vi "AlliGator Load Piccolo hist .bin Data.vi"(4 "# Pixels Y":i32, 6 "# Pixels X":i32, 8 "error in (no error)":errorcluster, 9 "# TCSPC Bins":i32, 11 "path in":path) -> (0 "error out":errorcluster, 2 "Array":u16[][][](array[numeric]), 3 "path out":path)   [LabVIEW 2021, in "AlliGator Files.lvlib"]
doc: "Loads Piccolo binned data."
uses:
  AlliGator Files.lvlib
panel:
  # "see the AlliGator License on the block diagram (Ctrl+E or Window:Show Block Diagram)"
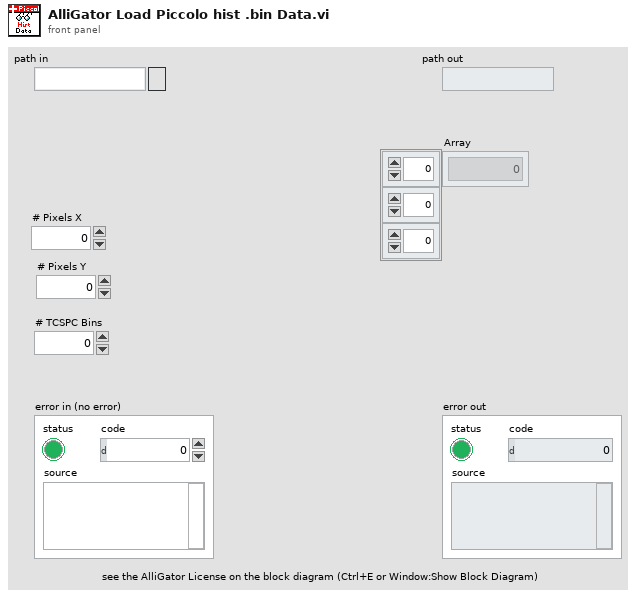
[diagram p1: front panel]
types:
  T1 = enum16{"big-endian, network order", "native, host order", "little-endian"}
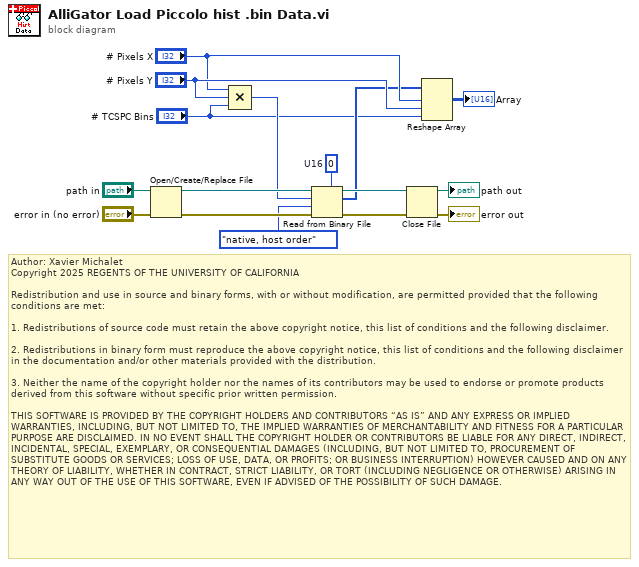
[diagram p0: block diagram]
diagram:
  w7 = u16 0  # U16
  # "Author: Xavier Michalet\nCopyright 2025 REGENTS OF THE UNIVERSITY OF CALIFORNIA\n\nRedistribution and use in source and binary forms, with or without modification, are permitted provided that the following conditions are met:\n\n1. Redistributions of source code must retain the above copyright notice, this list of conditions and the following disclaimer.\n\n2. Redistributions in binary form must reproduce the above copyright notice, this list of conditions and the following disclaimer in the documentation and/or other materials provided with the distribution.\n\n3. Neither the name of the copyright holder nor the names of its contributors may be used to endorse or promote products derived from this software without specific prior written permission.\n\nTHIS SOFTWARE IS PROVIDED BY THE COPYRIGHT HOLDERS AND CONTRIBUTORS “AS IS” AND ANY EXPRESS OR IMPLIED WARRANTIES, INCLUDING, BUT NOT LIMITED TO, THE IMPLIED WARRANTIES OF MERCHANTABILITY AND FITNESS FOR A PARTICULAR PURPOSE ARE DISCLAIMED. IN NO EVENT SHALL THE COPYRIGHT HOLDER OR CONTRIBUTORS BE LIABLE FOR ANY DIRECT, INDIRECT, INCIDENTAL, SPECIAL, EXEMPLARY, OR CONSEQUENTIAL DAMAGES (INCLUDING, BUT NOT LIMITED TO, PROCUREMENT OF SUBSTITUTE GOODS OR SERVICES; LOSS OF USE, DATA, OR PROFITS; OR BUSINESS INTERRUPTION) HOWEVER CAUSED AND ON ANY THEORY OF LIABILITY, WHETHER IN CONTRACT, STRICT LIABILITY, OR TORT (INCLUDING NEGLIGENCE OR OTHERWISE) ARISING IN ANY WAY OUT OF THE USE OF THIS SOFTWARE, EVEN IF ADVISED OF THE POSSIBILITY OF SUCH DAMAGE."
  n1 = Open/Create/Replace File(file path (use dialog)="path in", error in="error in (no error)") -> (refnum out=w13:refnum<file>, error out=w14:errorcluster)  [unwired: 4 in, 1 out]
  n2 = Compound Arithmetic op=MULTIPLY("# Pixels X", "# Pixels Y", "# TCSPC Bins") -> (w4:i32)
  n3 = Read from Binary File(5:w7, 8:w14, 9:T1."native, host order" ("byte order (0:big-endian, network order)"), 10:w4, 11:w13) -> (0:w2:errorcluster, 2:w5:u16[], 3:w15:refnum<file>)  [unwired: 1 in, 1 out]
  n4 = Close File(refnum=w15, error in=w2) -> (path=→"path out":path, error out=→"error out":errorcluster)
  n5 = Reshape Array(w5, "# Pixels X", "# Pixels Y", "# TCSPC Bins") -> (→"Array":u16[][][])
